vi "Read Inputs from system.vi"(8 "error in":errorcluster, 11 "State Machine runtime in":refnum<class "State Machine runtime.lvclass">) -> (0 "error out":errorcluster, 2 "Inputs from system":T1, 3 "State Machine runtime out":refnum<class "State Machine runtime.lvclass">)   [LabVIEW 2021, in "State Machine runtime.lvclass"]
uses:
  State Machine runtime.lvclass
  configuration/input data indices.ctl
  State Machine runtime.lvclass/State Machine runtime.ctl
  configuration/State Machine configuration.lvclass
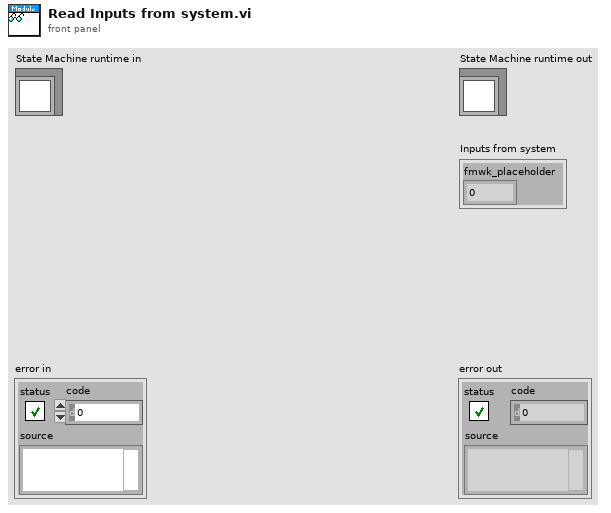
[diagram p1: front panel]
types:
  T1 = typedef "State Machine configuration.lvclass/input data indices.ctl" = cluster{"fmwk_placeholder":i32}
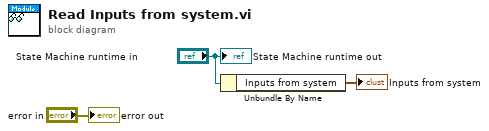
[diagram p0: block diagram]
diagram:
  n1 = Unbundle By Name("State Machine runtime in") -> ("Inputs from system"=→"Inputs from system":T1)
  "error out" <- "error in"
  "State Machine runtime out" <- "State Machine runtime in"
